vi "Pre Launch Init.vi"(11 "Zen Analytics.lvlib:Zen Analytics.lvclass":refnum<class "Zen Analytics.lvclass">) -> (0 "error out":errorcluster, 3 "Zen Analytics.lvlib:Zen Analytics.lvclass 2":refnum<class "Zen Analytics.lvclass">)   [LabVIEW 2019, in "Zen Analytics.lvlib" / "Zen Analytics.lvclass"]
doc: "(<B>Filename</B>: Actor Framework.lvlib:Actor.lvclass:Pre Launch Init.vi)\n\nDefines behavior that occurs after the Launch Nested Actor method is invoked but before the actor's Actor Core method begins running.\n\nBy default, this method does nothing. A descendant class may override it to define behavior."
uses:
  Zen Analytics.lvclass
  <vilib>/ActorFramework/Actor/Actor.lvclass
  Dependency/InterDataCommunication.ctl
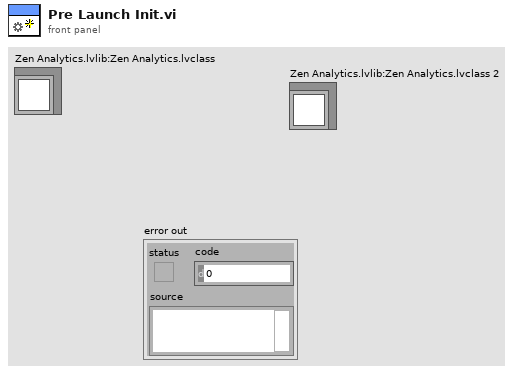
[diagram p1: front panel]
types:
  T1 = typedef "Zen Analytics.lvlib/Zen Analytics.lvclass/InterDataCommunication.ctl" = cluster{"State Name":string, "Data":variant}
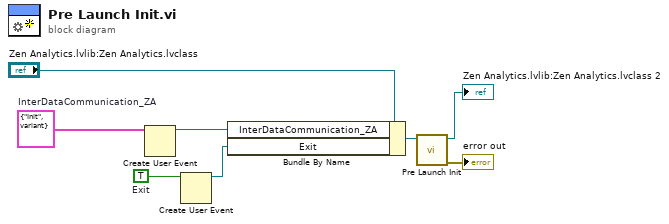
[diagram p0: block diagram]
diagram:
  w6 = T1 {"State Name"="Init", "Data"=variant}  # InterDataCommunication_ZA
  w7 = TRUE  # Exit
  n1 = Create User Event(user event datatype=w6) -> (user event=w5:refnum<user-event>)  [unwired: 1 in, 1 out]
  n2 = Create User Event(user event datatype=w7) -> (user event=w1:refnum<user-event>)  [unwired: 1 in, 1 out]
  n3 = Bundle By Name(cluster="Zen Analytics.lvlib:Zen Analytics.lvclass", "InterDataCommunication_ZA"=w5, "Exit"=w1) -> (w4:refnum<class "Zen Analytics.lvclass">)
  n4 = call-parent "Pre Launch Init.vi"("Actor in"=w4) -> ("error out"=→"error out":errorcluster, "Actor out"=→"Zen Analytics.lvlib:Zen Analytics.lvclass 2":refnum<class "Zen Analytics.lvclass">)  [unwired: 9 in]
